vi "Cont Acq&Graph Voltage-Int Clk_mod.vi"() -> ()   [LabVIEW 2010]
doc: "I. Description:\nThis example demonstrates how to acquire a continuous amount of data (Waveform) using the DAQ device's internal clock.\n\nII. Instructions for Running:\n1. Select the physical channel to correspond to where your signal is input on the DAQ device.\n2. Enter the minimum and maximum voltages.\nNote: For better accuracy try to match the input range to the expected voltage level of the measured signal.\n3. Select the number of samples to acquire per loop iteration.\n4. Set the rate of the acquisition\nNote: The rate should be AT LEAST twice as fast as the maximum frequency component of the signal being acquired.\n\nIII. Block Diagram Steps:\n1. Create an analog input voltage channel.\n2. Set the rate for the sample clock. Additionally, define the sample mode to be continuous.\n3. Call the Start VI to start the acquisition.\n4. Read the waveform data in a loop until the user hits the stop button or an error occurs.\nNote: This example reads data from one or more channels and returns an array of data. Use the Index Array function to access an individual channel of data.\n5. Call the Clear Task VI to clear the Task.\n6. Use the popup dialog box to display an error if any.\n\nIV. I/O Connections Overview:\nMake sure your signal input terminal matches the Physical Channel I/O Control. For further connection information, refer to your hardware reference manual."
uses:
  <vilib>/Utility/error.llb/DialogType.ctl
  <vilib>/DAQmx/read.llb/DAQmx Read (Analog 1D Wfm NChan NSamp).vi
  <vilib>/daqmx/miscellaneous.llb/DAQmx Fill In Error Info.vi
panel:
  in  "Physical Channel":tag="Dev1/ai0"
  in  "stop":bool
  in  "Sample Rate":dbl=10000.0 caption="Sample Rate (Hz)" format="%0.2f"
  out "Graph":waveform(dbl)[](graph) caption="Measurement"
  # "Channel Parameters"
  # "Timing Parameters"
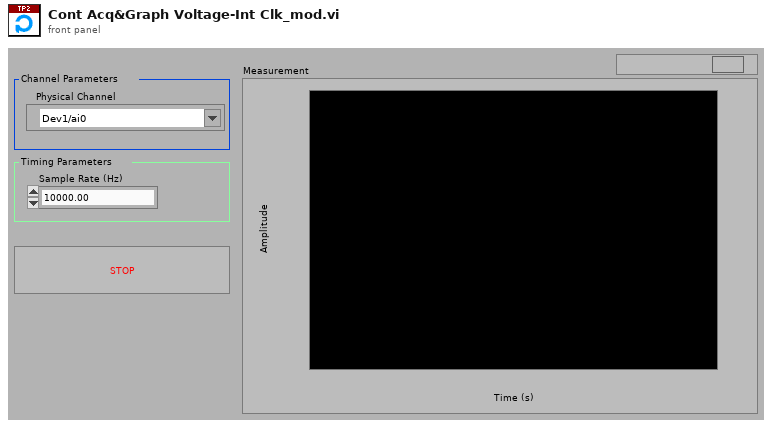
[diagram p1: front panel]
types:
  T1 = typedef "DialogType.ctl" = u16
  T2 = cluster{"file format":string, "Application Directory":path, "tdms":refnum<k34>}
  T3 = enum32{"invalid app kind", "Development System", "Run Time System", "Student Edition", "Embedded LabVIEW", "Evaluation", "Custom"}
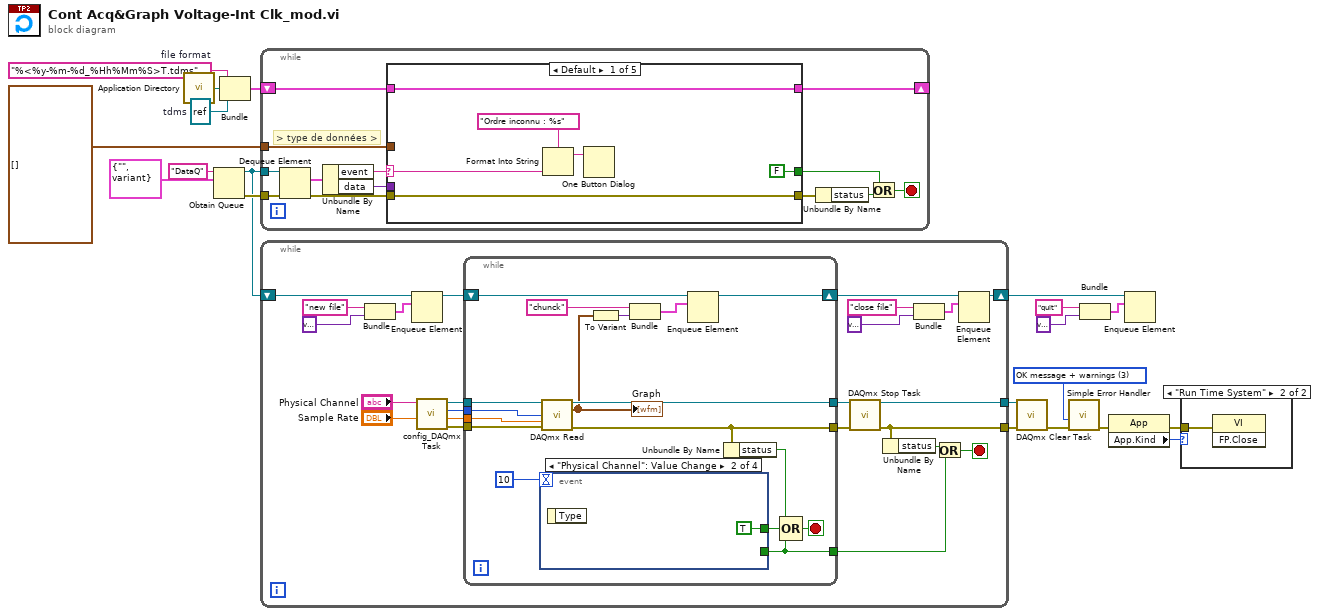
[diagram p0: block diagram]
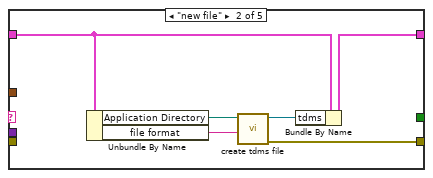
[diagram p2: hidden frame]
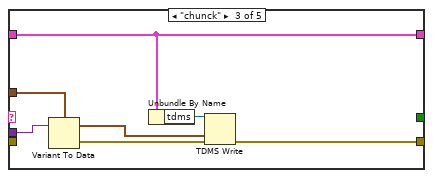
[diagram p3: hidden frame]
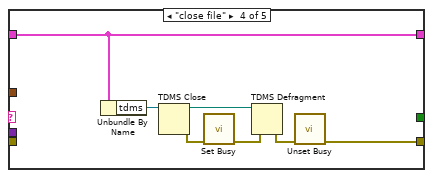
[diagram p4: hidden frame]
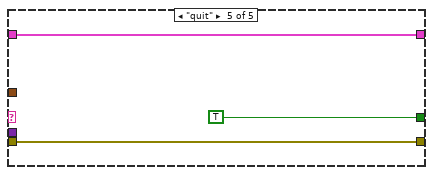
[diagram p5: hidden frame]
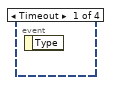
[diagram p7: hidden frame]
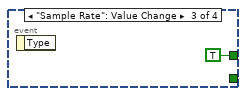
[diagram p8: hidden frame]
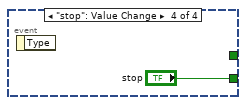
[diagram p9: hidden frame]
diagram:
  w7 = "%<%y-%m-%d_%Hh%Mm%S>T.tdms"  # file format
  w6 = refnum<k34> refnum  # tdms
  w19 = T1 3 items=["no dialog", "OK message", "continue or stop message", "OK message + warnings", "continue/stop + warnings"] ("type of dialog (OK msg:1)")
  n1 = call <vilib>:"Application Directory.vi"() -> ("Application Directory"=w9:path)
  n2 = Obtain Queue(name (unnamed)="DataQ", element data type=cluster{"event":string, "data":variant} {"event"="", "data"=variant}) -> (queue out=w10:refnum<queue>, error out=w12:errorcluster)  [unwired: 3 in, 1 out]
  n3 = Bundle("file format"=w7, "Application Directory"=w9, "tdms"=w6) -> (w8:T2)  [unwired: 1 in]
  n4 = while {
    tunnel: w10 -> [w33]
    tunnel: w12 -> [w32]
    shift-right: [w27] -> _
    shift-left: w8 -> [w28]
    tunnel: waveform(dbl)[] [] -> [w21]
    stop <- w22 stop-if-true
    # "> type de données >"
    n5 = Dequeue Element(queue=w33, error in (no error)=w32) -> (element=w31:cluster{"event":string, "data":variant}, error out=w26:errorcluster)  [unwired: 1 in, 2 out]
    n6 = Unbundle By Name(w31) -> ("event"=w30:string, "data"=w29:variant)
    n7 = case shown="Default" w30 {
      selector: w30 -> [w35 _ _ _ _]
      tunnel: w29 -> [_ _ w50 _ _]
      tunnel: w28 -> [w39 w45 w51 w59 w62]
      tunnel: [w39 w44 w51 w59 w62] -> w27
      tunnel: [w38 w40 w49 w53 w61] -> w25
      tunnel: w26 -> [w38 _ _ _ w61]
      tunnel: [FALSE _ _ _ TRUE] -> w23
      tunnel: w21 -> [_ _ w48 _ _]
      frame Default {
        n8 = Format Into String(format string="Ordre inconnu : %s", w35) -> (resulting string=w36:string)  [unwired: 2 in, 1 out]
        n9 = One Button Dialog(message=w36) -> ()  [unwired: 1 in, 1 out]
      }
      frame "new file" {
        n10 = Unbundle By Name(w45) -> ("Application Directory"=w43:path, "file format"=w42:string)
        n11 = call "create tdms file.vi"("format"=w42, "Application Directory"=w43) -> ("error out"=w40:errorcluster, "tdms file out"=w41:refnum<k34>)  [unwired: 6 in]
        n12 = Bundle By Name(cluster=w45, "tdms"=w41) -> (w44:T2)
      }
      frame "chunck" {
        n13 = Variant To Data(Variant=w50, type=w48) -> (error out=w46:errorcluster, data=w47:waveform(dbl)[])  [unwired: 1 in]
        n14 = Unbundle By Name(w51) -> ("tdms"=w52:refnum<k34>)
        n15 = TDMS Write(0:w52, 9:w47, 11:w46) -> (15:w49:errorcluster)  [unwired: 3 in, 3 out]
      }
      frame "close file" {
        n16 = Unbundle By Name(w59) -> ("tdms"=w57:refnum<k34>)
        n17 = TDMS Close(11:w57) -> (0:w56:errorcluster, 3:w58:path)  [unwired: 1 in]
        n18 = call <vilib>:"Set Busy.vi"("error in (no error)"=w56) -> ("error out"=w55:errorcluster)  [unwired: 9 in, 1 out]
        n19 = TDMS Defragment(4:w55, 7:w58) -> (0:w54:errorcluster)
        n20 = call <vilib>:"Unset Busy.vi"("error in (no error)"=w54) -> ("error out"=w53:errorcluster)  [unwired: 10 in]
      }
      frame "quit" {
      }
    }
    n21 = Unbundle By Name(w25) -> ("status"=w24:bool)
    n22 = Or(x=w23, y=w24) -> (x .or. y?=w22:bool)
  }
  n23 = while {
    tunnel: [w82] -> w18
    tunnel: [w77] -> w17
    shift-right: [w63] -> w2
    shift-left: w10 -> [w70]
    stop <- w75 stop-if-true
    n24 = Bundle("new file", variant) -> (w71:cluster{string, variant})  [unwired: 1 in]
    n25 = Enqueue Element(queue=w70, element=w71) -> (queue out=w69:refnum<queue>)  [unwired: 2 in, 2 out]
    n26 = call "config_DAQmx Task.vi"("Sample Rate"="Sample Rate", "Physical Channel"="Physical Channel") -> ("error out"=w85:errorcluster, "timeout"=w78:dbl, "taille de bloc d'acquisition"=w79:i32, "task out"=w73:refnum<k21>)  [unwired: 4 in]
    n27 = while {
      tunnel: w85 -> [w102]
      tunnel: w73 -> [w101]
      tunnel: [w100] -> w84
      tunnel: [w86] -> w81
      tunnel: w79 -> [w97]
      tunnel: w78 -> [w96]
      tunnel: [w93] -> w74
      shift-right: [w87] -> w64
      shift-left: w69 -> [w92]
      stop <- w98 stop-if-true
      n28 = event shown="[1] \"Physical Channel\": Value Change" {
        selector: _ -> [_ _ _ _]
        dyn-events: _ -> [_ _ _ _]
        timeout: 10 -> [_ _ _ _]
        tunnel: [_ TRUE TRUE _] -> w94
        tunnel: [_ _ _ "stop"] -> w93
        event Timeout {
          n29 = event-data() -> ()  [unwired: 1 in, 1 out]
        }
        event "Physical Channel": Value Change {
          n30 = event-data() -> ()  [unwired: 1 in, 1 out]
        }
        event "Sample Rate": Value Change {
          n31 = event-data() -> ()  [unwired: 1 in, 1 out]
        }
        event "stop": Value Change {
          n32 = event-data() -> ()  [unwired: 1 in, 1 out]
        }
      }
      n33 = call-poly <vilib>:"DAQmx Read.vi"("task/channels in"=w101, "number of samples per channel"=w97, "timeout"=w96, "error in"=w102) -> ("task out"=w100:refnum<k21>, "data"=w89:waveform(dbl)[], "error out"=w86:errorcluster)  [unwired: 9 in]
      "Graph" <- w89
      n34 = To Variant(anything=w89) -> (Variant=w88:variant)
      n35 = Bundle("chunck", "Variant"=w88) -> (w91:cluster{string, "Variant":variant})  [unwired: 1 in]
      n36 = Enqueue Element(queue=w92, element=w91) -> (queue out=w87:refnum<queue>)  [unwired: 2 in, 2 out]
      n37 = Unbundle By Name(w86) -> ("status"=w99:bool)
      n38 = Compound Arithmetic op=OR(w99, w94, w93) -> (w98:bool)
    }
    n39 = call <vilib>:"DAQmx Stop Task.vi"("task/channels in"=w84, "error in"=w81) -> ("task out"=w82:refnum<k21>, "error out"=w77:errorcluster)  [unwired: 12 in]
    n40 = Unbundle By Name(w77) -> ("status"=w76:bool)
    n41 = Bundle("close file", variant) -> (w66:cluster{string, variant})  [unwired: 1 in]
    n42 = Or(x=w76, y=w74) -> (x .or. y?=w75:bool)
    n43 = Enqueue Element(queue=w64, element=w66) -> (queue out=w63:refnum<queue>)  [unwired: 2 in, 2 out]
  }
  n44 = call <vilib>:"DAQmx Clear Task.vi"("task in"=w18, "error in"=w17) -> ("error out"=w20:errorcluster)  [unwired: 13 in]
  n45 = call <vilib>:"Simple Error Handler.vi"("type of dialog (OK msg:1)"=w19, "error in (no error)"=w20) -> ("error out"=w16:errorcluster)  [unwired: 3 in, 4 out]
  n46 = Bundle("quit", variant) -> (w4:cluster{string, variant})  [unwired: 1 in]
  n47 = property class="App"(error in=w16) -> (error out=w15:errorcluster, "App.Kind"=w14:T3)  [unwired: 1 in, 1 out]
  n48 = Enqueue Element(queue=w2, element=w4) -> ()  [unwired: 2 in, 3 out]
  n49 = case shown="\"Run Time System\"" w14 {
    tunnel: w15 -> [_ w106]
    frame Default {
    }
    frame "Run Time System" {
      n50 = invoke class="VI" method="FP.Close"(error in=w106) -> ()  [unwired: 2 in, 3 out]
    }
  }
